vi "Startup.vi"(6 "LabVIEW Web Service":refnum<class "Web Service.lvclass">) -> ()   [LabVIEW 2019]
uses:
  <vilib>/wsapi/Web Service.lvclass
panel:
  out "element":string
  out "Waveform Viewer":dbl[][](graph)
  # "Use the web service input terminal to call the VIs on the Service subpalette of the Web Services palette. Do not remove it from the connector pane unless you don't need access to the palette."
  # "Any additional terminals added to the connector pane of a startup VI will be ignored."
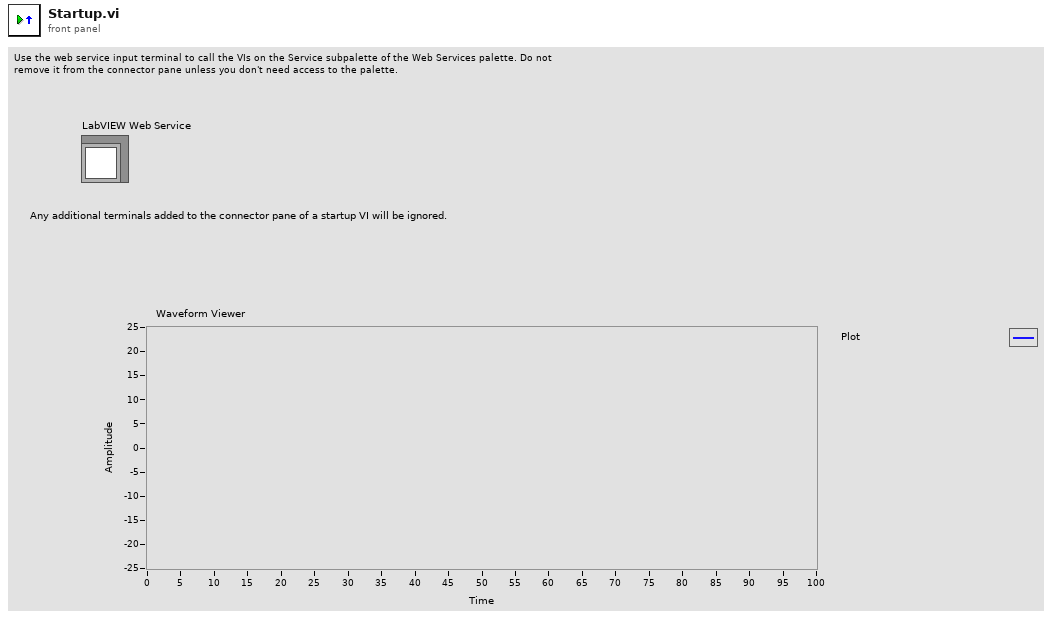
[diagram p1: front panel]
types:
  T1 = cluster{"name":string, "source":string, "value":dbl[]}[]
  T2 = cluster{"name":string, "value":dbl[], "source":string}[]
  T3 = cluster{"name":string, "source":string, "value":dbl[]}
  T4 = cluster{"name":string, "value":dbl[], "source":string}
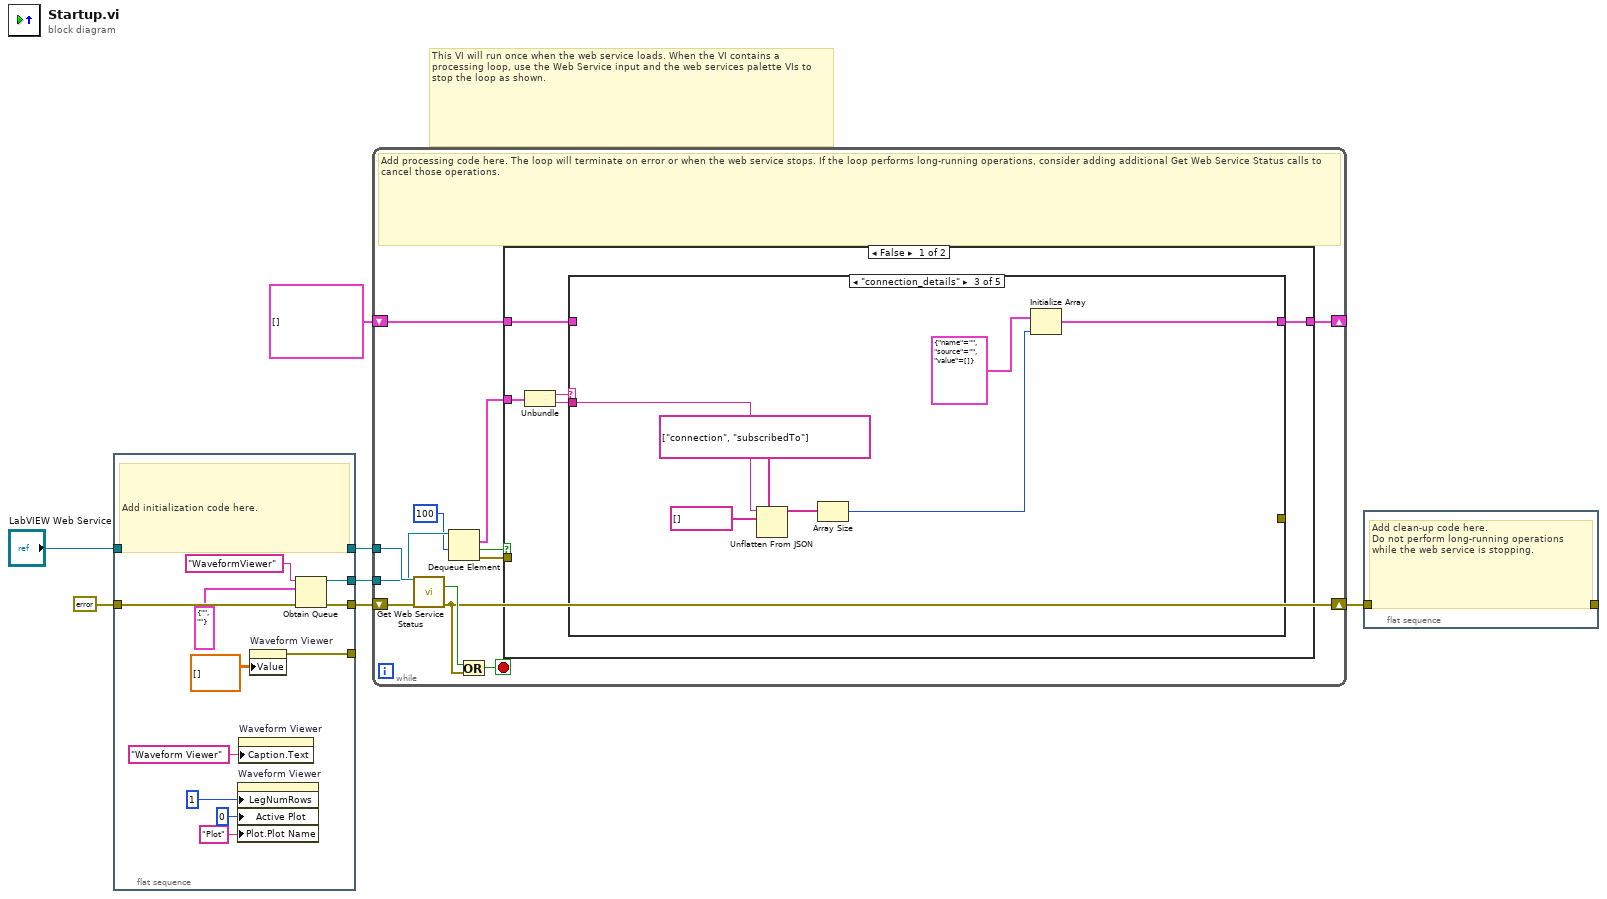
[diagram p0: block diagram]
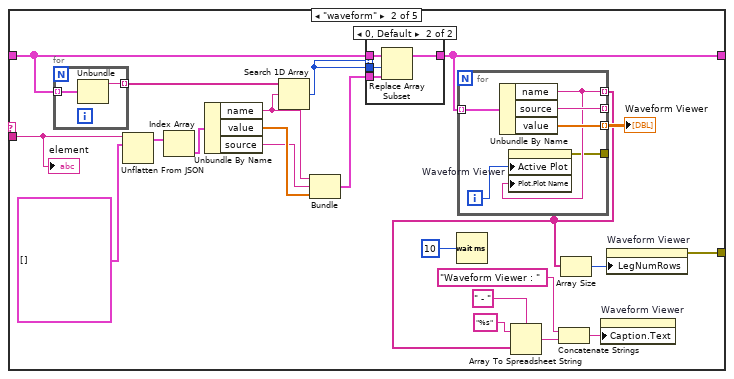
[diagram p3: hidden frame]
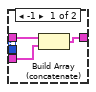
[diagram p4: hidden frame]
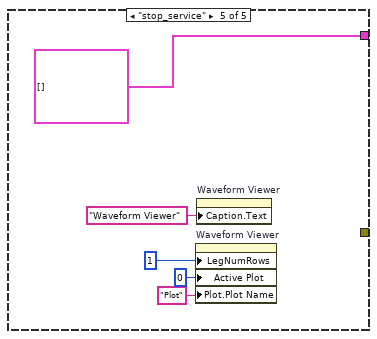
[diagram p6: hidden frame]
diagram:
  # "This VI will run once when the web service loads. When the VI contains a processing loop, use the Web Service input and the web services palette VIs to stop the loop as shown."
  n1 = flat-sequence {
    tunnel: "LabVIEW Web Service" -> [w19]
    tunnel: [w19] -> w6
    tunnel: [w18] -> w5
    tunnel: errorcluster {"status"=FALSE, "code"=0, "source"=""} ("error constant") -> [w17]
    tunnel: [w15] -> w2
    tunnel: [w13] -> _
    frame #0 {
      # "Add initialization code here."
      n2 = property on="Waveform Viewer" class="WFGraph (strict)"("LegNumRows"=u32 1 ("Legend:Number of Rows"), "Active Plot"=u32 0, "Plot.Plot Name"="Plot") -> ()  [unwired: 2 in, 2 out]
      n3 = property on="Waveform Viewer" class="WFGraph (strict)"("Caption.Text"="Waveform Viewer") -> ()  [unwired: 2 in, 2 out]
      n4 = property on="Waveform Viewer" class="WFGraph (strict)"("Value"=dbl[][] [] ("Waveform Viewer")) -> (error out=w13:errorcluster)  [unwired: 2 in, 1 out]
      n5 = Obtain Queue(name (unnamed)="WaveformViewer", element data type=cluster{string, "postdata":string} {"", "postdata"=""} ("output cluster"), error in (no error)=w17) -> (queue out=w15:refnum<queue>, error out=w18:errorcluster)  [unwired: 2 in, 1 out]
    }
  }
  n6 = while {
    tunnel: w6 -> [w30]
    shift-right: [w27] -> w3
    shift-left: w5 -> [w28]
    tunnel: w2 -> [w26]
    shift-right: [w21] -> _
    shift-left: T1 [] -> [w20]
    stop <- w29 stop-if-true
    # "Add processing code here. The loop will terminate on error or when the web service stops. If the loop performs long-running operations, consider adding additional Get Web Service Status calls to cancel those operations."
    n7 = call <vilib>:"Get Web Service Status.vi"("LabVIEW Web Service"=w30, "error in (no error)"=w28) -> ("service stopping?"=w31:bool, "error out"=w27:errorcluster)  [unwired: 11 in, 1 out]
    n8 = Dequeue Element(queue=w26, timeout in ms (-1)=100) -> (element=w22:cluster{string, "postdata":string}, timed out?=w24:bool, error out=w23:errorcluster)  [unwired: 1 in, 1 out]
    n9 = Or(x=w31, y=w27) -> (x .or. y?=w29:bool)
    n10 = case shown="False" w24 {
      tunnel: w23 -> [_ _]
      tunnel: w22 -> [w36 _]
      tunnel: [w33 w88] -> w21
      tunnel: w20 -> [w32 w88]
      frame False {
        n11 = Unbundle(w36) -> (w35:string, "postdata"=w34:string)
        n12 = case shown="\"connection_details\"" w35 {
          tunnel: w34 -> [_ w52 w81 _ _]
          tunnel: [w37 w42 w75 w82 T1 []] -> w33
          tunnel: w32 -> [w37 w45 _ w82 _]
          tunnel: [_ w38 _ _ _] -> _
          frame Default {
          }
          frame "waveform" {
            n13 = for {
              tunnel: w45 -> [w74] mode=indexing
              tunnel: [w73] -> w47 mode=indexing
              n14 = Unbundle(w74) -> ("name"=w73:string)  [unwired: 2 out]
            }
            n15 = Unflatten From JSON(JSON string=w52, type and defaults=T2 []) -> (value=w50:T2)  [unwired: 5 in, 1 out]
            n16 = Index Array(array=w50) -> (element=w49:T4)  [unwired: 1 in]
            n17 = Unbundle By Name(w49) -> ("name"=w46:string, "value"=w51:dbl[], "source"=w48:string)
            n18 = Search 1D Array(1D array=w47, element=w46) -> (index of element=w43:i32)  [unwired: 1 in]
            n19 = Bundle("name"=w46, "source"=w48, "value"=w51) -> (w44:T3)  [unwired: 1 in]
            n20 = case shown="0, Default" w43 {
              tunnel: w45 -> [w68 w72]
              tunnel: w43 -> [_ w71]
              tunnel: w44 -> [w66 w70]
              tunnel: [w67 w69] -> w42
              frame -1 {
                n21 = Build Array (concatenate)(w68, w66) -> (w67:T1)
              }
              frame 0, Default {
                n22 = Replace Array Subset(array=w72, new element=w70, index=w71) -> (w69:T1)
              }
            }
            n23 = Wait (ms)(milliseconds to wait=u32 10) -> ()  [unwired: 1 out]
            n24 = for {
              tunnel: w42 -> [w65] mode=indexing
              tunnel: [w61] -> w39 mode=indexing
              tunnel: [w64] -> _ mode=indexing
              tunnel: [w63] -> w41 mode=indexing
              tunnel: [w60] -> _
              i -> [w62]
              n25 = Unbundle By Name(w65) -> ("name"=w61:string, "source"=w64:string, "value"=w63:dbl[])
              n26 = property on="Waveform Viewer" class="WFGraph (strict)"("Active Plot"=w62, "Plot.Plot Name"=w61) -> (error out=w60:errorcluster)  [unwired: 2 in, 1 out]
            }
            "Waveform Viewer" <- w41
            n27 = Array To Spreadsheet String(delimiter (Tab)=" - ", array=w39, 3:"%s" ("format string")) -> (spreadsheet string=w56:string)
            n28 = Concatenate Strings("Waveform Viewer : " ("string"), w56) -> (w57:string)
            n29 = Array Size(array=w39) -> (size(s)=w40:i32)
            n30 = property on="Waveform Viewer" class="WFGraph (strict)"("Caption.Text"=w57) -> ()  [unwired: 2 in, 2 out]
            n31 = property on="Waveform Viewer" class="WFGraph (strict)"("LegNumRows"=w40) -> (error out=w38:errorcluster)  [unwired: 2 in, 1 out]
            "element" <- w52
          }
          frame "connection_details" {
            n32 = Unflatten From JSON(path=string[] ["connection", "subscribedTo"], JSON string=w81, type and defaults=string[] [] ("path")) -> (value=w78:string[])  [unwired: 4 in, 1 out]
            n33 = Array Size(array=w78) -> (size(s)=w77:i32)
            n34 = Initialize Array(T3 {"name"="", "source"="", "value"=[]}, w77) -> (w75:T1)
          }
          frame "start_service" {
          }
          frame "stop_service" {
            n35 = property on="Waveform Viewer" class="WFGraph (strict)"("LegNumRows"=u32 1 ("Legend:Number of Rows"), "Active Plot"=u32 0, "Plot.Plot Name"="Plot") -> ()  [unwired: 2 in, 2 out]
            n36 = property on="Waveform Viewer" class="WFGraph (strict)"("Caption.Text"="Waveform Viewer") -> ()  [unwired: 2 in, 2 out]
          }
        }
      }
      frame True {
      }
    }
  }
  n37 = flat-sequence {
    tunnel: [w89] -> _
    tunnel: w3 -> [w89]
    frame #0 {
      # "Add clean-up code here.\nDo not perform long-running operations while the web service is stopping."
    }
  }
